vi "Part 1.vi"(11 "Input":string) -> (3 "Output":i64)   [LabVIEW 2021]
uses:
  <vilib>/regexp/Match Regular Expression.xnode
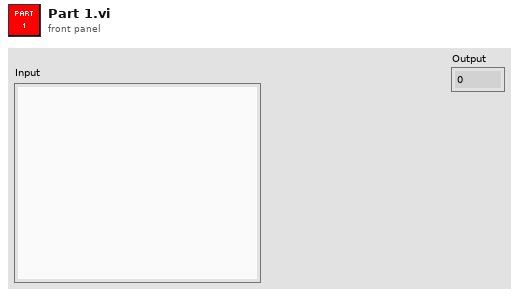
[diagram p1: front panel]
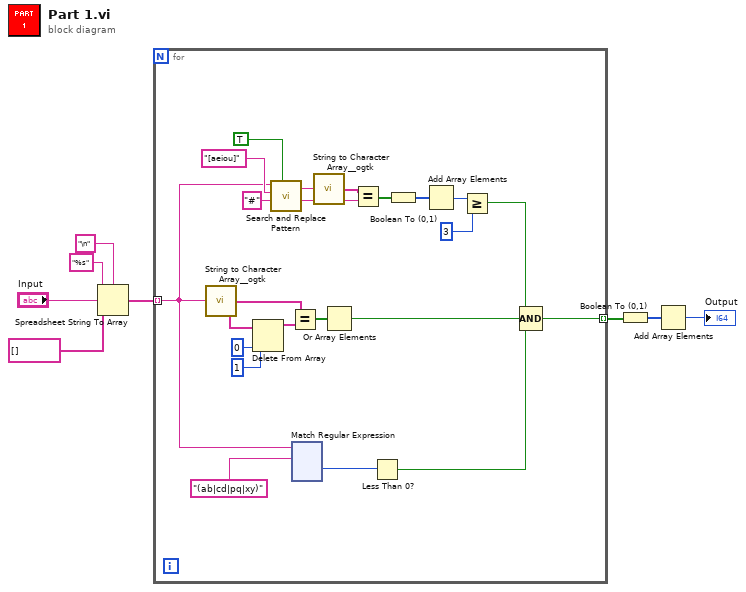
[diagram p0: block diagram]
diagram:
  n1 = Spreadsheet String To Array(delimiter (Tab)="\n", format string="%s", spreadsheet string="Input", array type (2D Dbl)=string[] []) -> (array=w4:string[])
  n2 = for {
    tunnel: w4 -> [w12] mode=indexing
    tunnel: [w13] -> w2 mode=indexing
    w21 = "#" ("replace string (\"\")")
    n3 = call <userlib>:"String to Character Array__ogtk.vi"("Input String"=w12) -> ("Character Array"=w26:string[])
    n4 = Delete From Array(array=w26, length=1, index=0) -> (array with subset deleted=w27:string[])  [unwired: 1 out]
    n5 = call <vilib>:"Search and Replace Pattern.vi"("string"=w12, "regular expression (\"\")"="[aeiou]" ("replace string (\"\")"), "replace string (\"\")"=w21, "replace all? (F)"=TRUE) -> ("result string"=w22:string)  [unwired: 1 in, 1 out]
    n6 = Equal?(x=w26, y=w27) -> (x = y?=w25:bool[])
    n7 = xnode "Match Regular Expression"("input string"=w12, "regular expression"="(ab|cd|pq|xy)" ("replace string (\"\")")) -> ("offset past match"=w10:i32)  [unwired: 4 in, 4 out]
    n8 = call <userlib>:"String to Character Array__ogtk.vi"("Input String"=w22) -> ("Character Array"=w20:string[])
    n9 = Or Array Elements(Boolean array=w25) -> (logical OR=w14:bool)
    n10 = Equal?(x=w20, y=w21) -> (x = y?=w19:bool[])
    n11 = Less Than 0?(x=w10) -> (x < 0?=w9:bool)
    n12 = Boolean To (0,1)(Boolean=w19) -> (0, 1=w18:i16[])
    n13 = Add Array Elements(numeric array=w18) -> (sum=w17:i16)
    n14 = Greater Or Equal?(x=w17, y=i16 3) -> (x >= y?=w15:bool)
    n15 = Compound Arithmetic op=AND(w15, w14, w9) -> (w13:bool)
  }
  n16 = Boolean To (0,1)(Boolean=w2) -> (0, 1=w3:i16[])
  n17 = Add Array Elements(numeric array=w3) -> (sum=→"Output":i16)
